vi "Input File Mode State Machine.vi"(0 "Mixed Mode Widget Requests":T9, 1 "MM In":refnum<queue>, 2 "Mixed Mode Command In":T2, 5 "Mixed Mode Widget Actions In":T8, 7 "Mixed Mode Blinkies In":T7, 13 "MixedModeStates In":T1=enum."Idle") -> (4 "Mixed Mode Widget Approval":T9, 6 "Mixed Mode Widget Actions Out":T8, 8 "Mixed Mode Blinkies Out":T7, 12 "MM Out":refnum<queue>)   [LabVIEW 2009]
uses:
  Mixed Mode Widget Requests.ctl
  Accepted or Declined.ctl
  Mixed Mode Widget State.ctl
  Messages/Mixed Mode Command.ctl
  Mixed Mode Command Action.ctl
  Ramp Time Tuple.ctl
  Target Data.ctl
  Data Access Objects/Metadata/LBCB Space.ctl
  Mixed Mode Blinkies.ctl
  Mixed Mode States.ctl
  Target Pattern.ctl
  Step DAO Actions.ctl
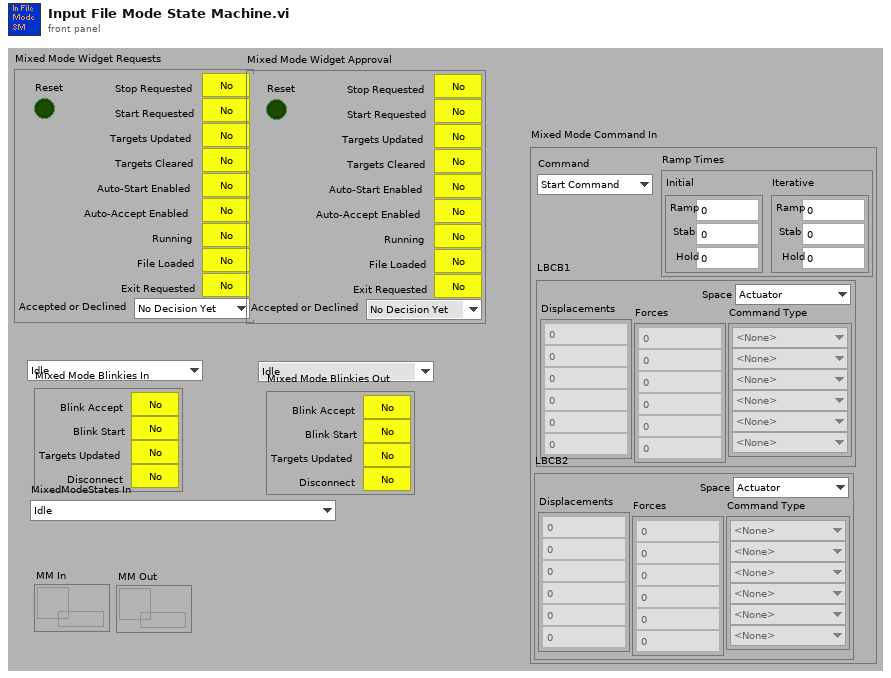
[diagram p1: front panel]
types:
  T1 = typedef "Mixed Mode States.ctl" = enum16{"Init", "Wait For DAQ", "Idle", "Start Initial Position", "Initial Position", "Start Initial Ramp", "Run Initial Ramp", "Start Iterative Stage", "Convergence Check", "Update Stiffness Jacobian", "Update Command", "Start Iterative Ramp", "Run Iterative Ramp", "Start Iterative Stabilize", "Iterative Stabilize", "Start Iterative Holding", "Iterative Holding", "Start Stabilize", "Stabilize", "Start Hold", "Holding", "Done", "Aborting", "Exit", "Nop"}
  T2 = typedef "Mixed Mode Command.ctl" = cluster{"Command":T3, "Ramp Times":cluster{"Initial":T4, "Iterative":T4}, "LBCB1":T5, "LBCB2":T5}
  T3 = typedef "Mixed Mode Command Action.ctl" = enum16{"Start Command", "Stop", "Exit", "No Op", "Start Acquisition", "Measure Initial Position"}
  T4 = typedef "Ramp Time Tuple.ctl" = cluster{"Ramp":dbl, "Stab":dbl, "Hold":dbl}
  T5 = typedef "Target Data.ctl" = cluster{"Displacements":dbl[], "Command Type":enum16{"<None>", "Displacement", "Force"}[], "Forces":dbl[], "Space":T6}
  T6 = typedef "LBCB Space.ctl" = enum16{"Actuator", "Cartesian"}
  T7 = typedef "Mixed Mode Blinkies.ctl" = cluster{"Blink Accept":bool, "Blink Start":bool, "Targets Updated":bool, "Disconnect":bool}
  T8 = typedef "Mixed Mode Widget State.ctl" = enum16{"Idle", "Auto Start", "Wait for Start", "Start", "Wait for Hold", "Waiting for Done", "Step Completed", "Limit Fault", "Stop", "Abort", "Clear Targets", "Reset", "Steps Loaded", "Paused", "Steps Available", "Load Step", "Connected", "Disconnecting", "Wait for Proposal", "Auto Accept", "Wait for Accept", "Accept", "Decline", "Wait for Execute", "Unknown", "Exit"}
  T9 = typedef "Mixed Mode Widget Requests.ctl" = cluster{"Start Requested":bool, "Targets Updated":bool, "Targets Cleared":bool, "Stop Requested":bool, "Auto-Start Enabled":bool, "Auto-Accept Enabled":bool, "Accepted or Declined":T10, "Running":bool, "File Loaded":bool, "Reset":bool, "Exit Requested":bool}
  T10 = typedef "Accepted or Declined.ctl" = enum16{"No Decision Yet", "Accepted", "Declined"}
  T11 = typedef "Target Pattern.ctl" = enum16{"Clear Targets", "Reset Targets to Zero", "Displacements Only", "Rotations Only", "Displacements & Rotations", "Forces Only", "Moments Only", "Forces & Moments"}
  T12 = typedef "Step DAO Actions.ctl" = enum16{"Init", "Set", "Get", "Reset Count"}
  T13 = typedef "Target.ctl" = cluster{"LBCB Number":T14, "DOF Vectors":enum16{" ", "Dx", "Dy", "Dz", "Rx", "Ry", "Rz", "Fx", "Fy", "Fz", "Mx", "My", "Mz"}, "Amount":dbl}
  T14 = typedef "LBCB Number.ctl" = enum16{"LBCB1", "LBCB2"}
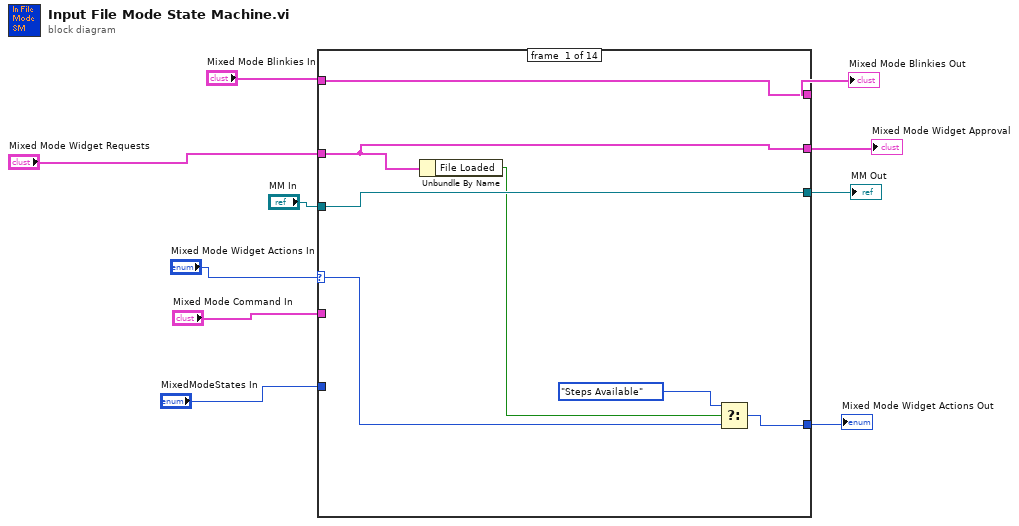
[diagram p0: block diagram]
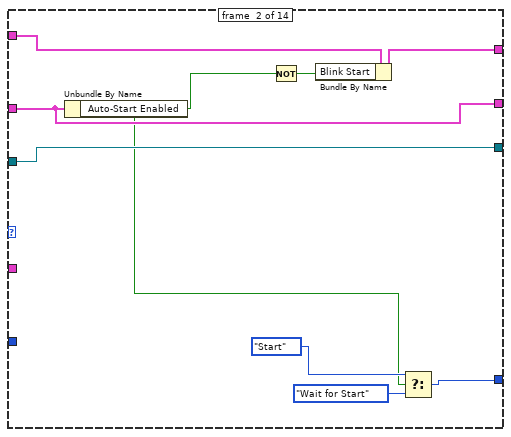
[diagram p2: hidden frame]
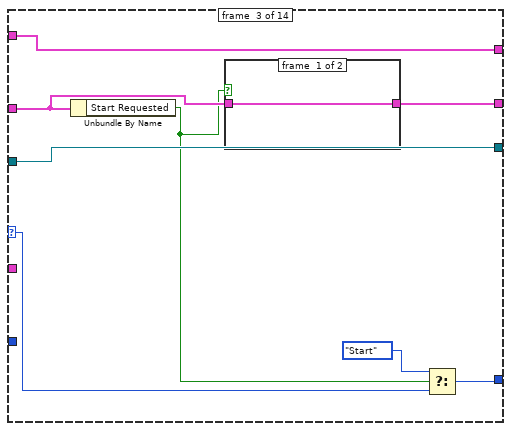
[diagram p3: hidden frame]
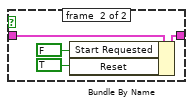
[diagram p4: hidden frame]
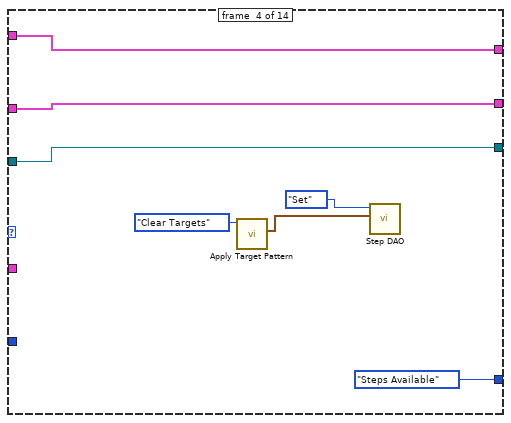
[diagram p5: hidden frame]
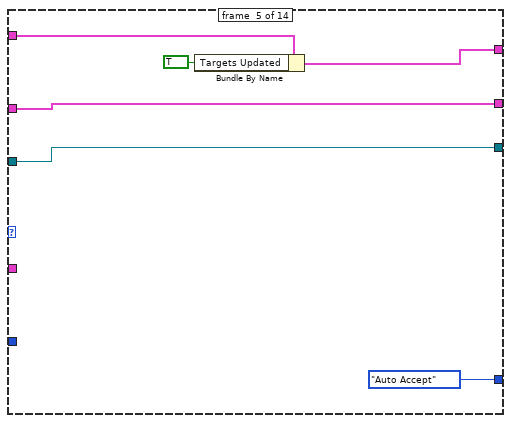
[diagram p6: hidden frame]
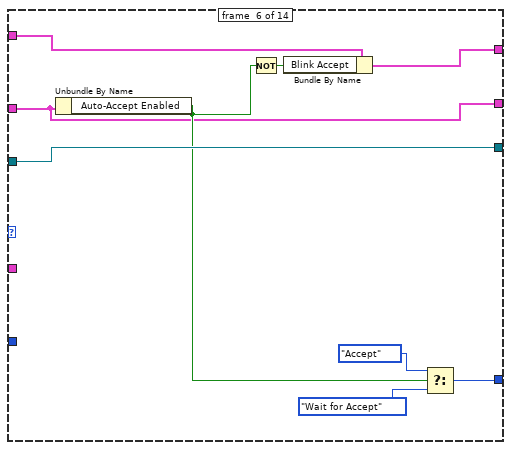
[diagram p7: hidden frame]
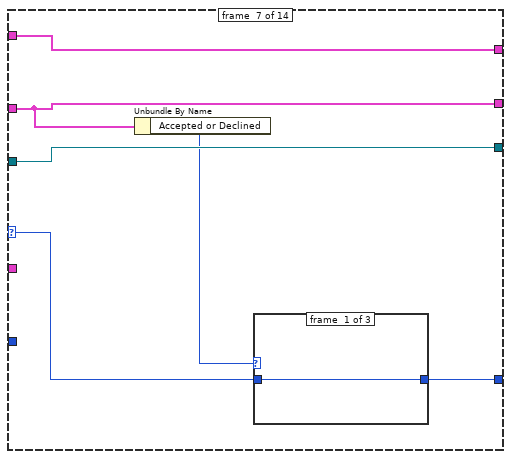
[diagram p8: hidden frame]
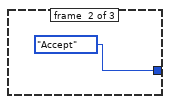
[diagram p9: hidden frame]
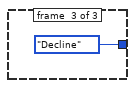
[diagram p10: hidden frame]
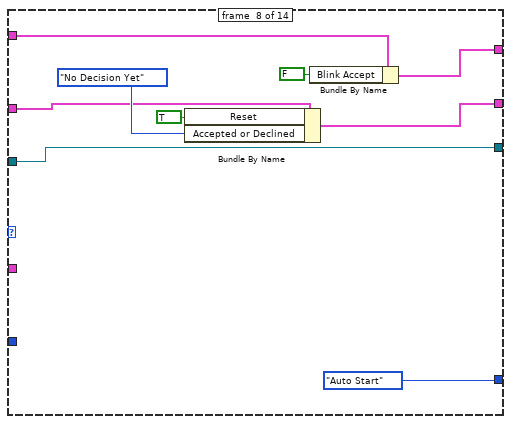
[diagram p11: hidden frame]
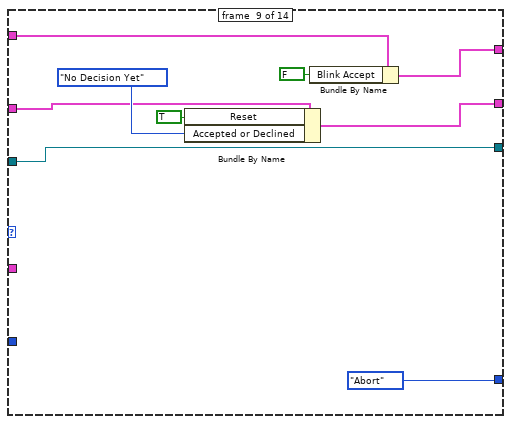
[diagram p12: hidden frame]
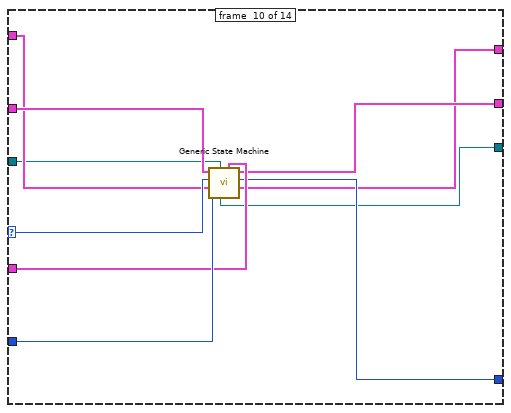
[diagram p13: hidden frame]
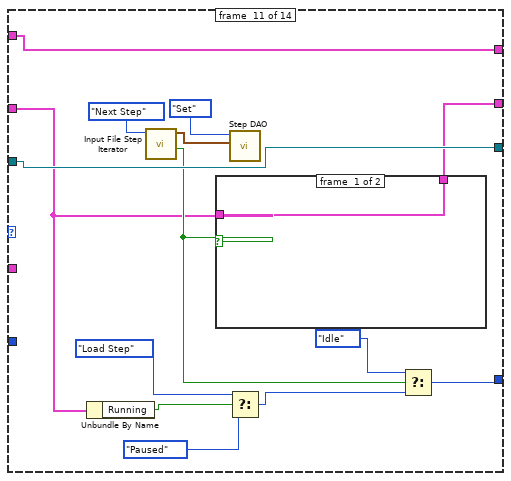
[diagram p14: hidden frame]
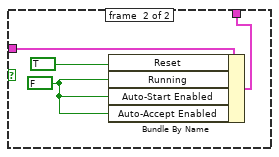
[diagram p15: hidden frame]
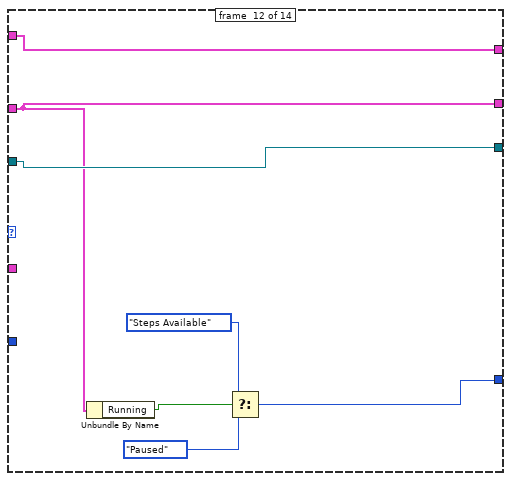
[diagram p16: hidden frame]
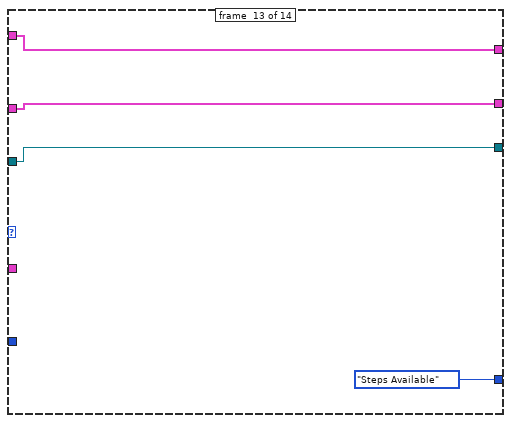
[diagram p17: hidden frame]
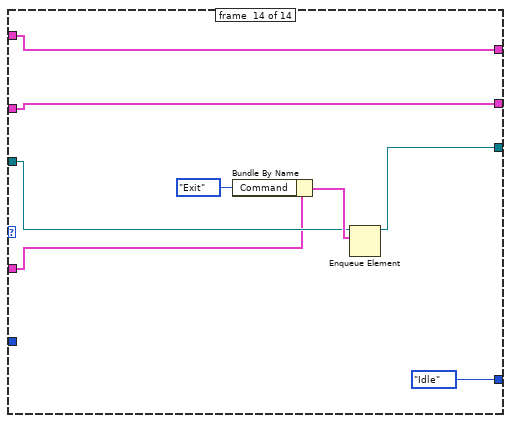
[diagram p18: hidden frame]
diagram:
  n1 = case shown="\"Steps Available\"" "Mixed Mode Widget Actions In" {
    selector: "Mixed Mode Widget Actions In" -> [w14 _ w27 _ _ _ w63 _ _ w97 _ _ _ _]
    tunnel: "Mixed Mode Widget Requests" -> [w12 w23 w30 w42 w52 w53 w62 w75 w84 w98 w100 w122 w127 w133]
    tunnel: "Mixed Mode Blinkies In" -> [w17 w26 w31 w43 w50 w61 w67 w79 w88 w96 w108 w124 w128 w134]
    tunnel: [w17 w25 w31 w43 w49 w56 w67 w78 w87 w90 w108 w124 w128 w134] -> w8
    tunnel: [w16 w20 w34 Mixed_Mode_Widget_State."Steps Available" ("Mixed Mode Widget Actions In") Mixed_Mode_Widget_State."Auto Accept" ("Mixed Mode Widget Actions In") w59 w64 Mixed_Mode_Widget_State."Auto Start" ("f") Mixed_Mode_Widget_State."Abort" ("f") w91 w109 w118 Mixed_Mode_Widget_State."Steps Available" ("f") Mixed_Mode_Widget_State."Idle" ("f")] -> w1
    tunnel: [w12 w23 w29 w42 w52 w53 w62 w74 w83 w92 w99 w122 w127 w133] -> w7
    tunnel: "Mixed Mode Command In" -> [_ _ _ _ _ _ _ _ _ w93 _ _ _ w130]
    tunnel: "MM In" -> [w13 w22 w32 w41 w51 w60 w66 w73 w82 w94 w107 w123 w126 w132]
    tunnel: [w13 w22 w32 w41 w51 w60 w66 w73 w82 w89 w107 w123 w126 w131] -> w4
    tunnel: "MixedModeStates In" -> [_ _ _ _ _ _ _ _ _ w95 _ _ _ _]
    frame #0 {
      n2 = Unbundle By Name(w12) -> ("File Loaded"=w11:bool)
      n3 = Select(t=Mixed_Mode_Widget_State."Steps Available" ("Mixed Mode Widget Actions In"), s=w11, f=w14) -> (s? t:f=w16:T8)
    }
    frame #1 {
      n4 = Unbundle By Name(w23) -> ("Auto-Start Enabled"=w19:bool)
      n5 = Not(x=w19) -> (.not. x?=w24:bool)
      n6 = Bundle By Name(cluster=w26, "Blink Start"=w24) -> (w25:T7)
      n7 = Select(t=Mixed_Mode_Widget_State."Start" ("Mixed Mode Widget Actions In"), s=w19, f=Mixed_Mode_Widget_State."Wait for Start") -> (s? t:f=w20:T8)
    }
    frame #2 {
      n8 = Unbundle By Name(w30) -> ("Start Requested"=w28:bool)
      n9 = case shown="False" w28 {
        tunnel: w30 -> [w35 w39]
        tunnel: [w35 w38] -> w29
        frame #0 {
        }
        frame #1 {
          n10 = Bundle By Name(cluster=w39, "Start Requested"=FALSE, "Reset"=TRUE) -> (w38:T9)
        }
      }
      n11 = Select(t=Mixed_Mode_Widget_State."Start", s=w28, f=w27) -> (s? t:f=w34:T8)
    }
    frame #3 {
      n12 = call "Apply Target Pattern.vi"("Target Pattern"=Target_Pattern."Clear Targets") -> ("Targets"=w45:T13[])  [unwired: 1 in, 9 out]
      n13 = call "Step DAO.vi"("Step In"=w45, "Step DAO Actions"=Step_DAO_Actions."Set") -> ()  [unwired: 2 in, 8 out]
    }
    frame #4 {
      n14 = Bundle By Name(cluster=w50, "Targets Updated"=TRUE) -> (w49:T7)
    }
    frame #5 {
      n15 = Unbundle By Name(w53) -> ("Auto-Accept Enabled"=w54:bool)
      n16 = Not(x=w54) -> (.not. x?=w55:bool)
      n17 = Bundle By Name(cluster=w61, "Blink Accept"=w55) -> (w56:T7)
      n18 = Select(t=Mixed_Mode_Widget_State."Accept" ("Mixed Mode Widget Actions In"), s=w54, f=Mixed_Mode_Widget_State."Wait for Accept") -> (s? t:f=w59:T8)
    }
    frame #6 {
      n19 = Unbundle By Name(w62) -> ("Accepted or Declined"=w65:T10)
      n20 = case shown="\"No Decision Yet\"" w65 {
        tunnel: [w68 Mixed_Mode_Widget_State."Accept" ("f") Mixed_Mode_Widget_State."Decline" ("f")] -> w64
        tunnel: w63 -> [w68 _ _]
        frame #0 {
        }
        frame #1 {
        }
        frame #2 {
        }
      }
    }
    frame #7 {
      n21 = Bundle By Name(cluster=w75, "Reset"=TRUE, "Accepted or Declined"=Accepted_or_Declined."No Decision Yet") -> (w74:T9)
      n22 = Bundle By Name(cluster=w79, "Blink Accept"=FALSE) -> (w78:T7)
    }
    frame #8 {
      n23 = Bundle By Name(cluster=w84, "Reset"=TRUE, "Accepted or Declined"=Accepted_or_Declined."No Decision Yet") -> (w83:T9)
      n24 = Bundle By Name(cluster=w88, "Blink Accept"=FALSE) -> (w87:T7)
    }
    frame #9 {
      n25 = call "Generic State Machine.vi"("Mixed Mode Command In"=w93, "MM In"=w94, "MixedModeStates In"=w95, "Mixed Mode Blinkies In"=w96, "Mixed Mode Widget Actions In"=w97, "Mixed Mode Widget Requests"=w98) -> ("Mixed Mode Blinkies Out"=w90:T7, "Mixed Mode Widget Actions Out"=w91:T8, "Mixed Mode Widget Approval"=w92:T9, "MM Out"=w89:refnum<queue>)  [unwired: 2 out]
    }
    frame #10 {
      n26 = Unbundle By Name(w100) -> ("Running"=w105:bool)
      n27 = call "Input File Step Iterator.vi"("Input File Step Actions"=enum16{"Load", "Next Step", "Reset"}."Next Step") -> ("End of Input File"=w101:bool, "Next Step"=w111:T13[])  [unwired: 3 in, 6 out]
      n28 = case shown="True" w101 {
        tunnel: w100 -> [w113 w117]
        tunnel: [w113 w116] -> w99
        frame #0 {
        }
        frame #1 {
          w114 = FALSE ("File Loaded")
          n29 = Bundle By Name(cluster=w117, "Reset"=TRUE, "Running"=w114, "Auto-Start Enabled"=w114, "Auto-Accept Enabled"=w114) -> (w116:T9)
        }
      }
      n30 = call "Step DAO.vi"("Step In"=w111, "Step DAO Actions"=Step_DAO_Actions."Set") -> ()  [unwired: 2 in, 8 out]
      n31 = Select(t=Mixed_Mode_Widget_State."Load Step" ("Mixed Mode Widget Actions In"), s=w105, f=Mixed_Mode_Widget_State."Paused") -> (s? t:f=w104:T8)
      n32 = Select(t=Mixed_Mode_Widget_State."Idle" ("f"), s=w101, f=w104) -> (s? t:f=w109:T8)
    }
    frame #11 {
      n33 = Unbundle By Name(w122) -> ("Running"=w120:bool)
      n34 = Select(t=Mixed_Mode_Widget_State."Steps Available" ("Mixed Mode Widget Actions In"), s=w120, f=Mixed_Mode_Widget_State."Paused") -> (s? t:f=w118:T8)
    }
    frame #12 {
    }
    frame #13 {
      n35 = Bundle By Name(cluster=w130, "Command"=Mixed_Mode_Command_Action."Exit") -> (w136:T2)
      n36 = Enqueue Element(queue=w132, element=w136) -> (queue out=w131:refnum<queue>)  [unwired: 1 in, 3 out]
    }
  }
  "Mixed Mode Widget Approval" <- w7
  "Mixed Mode Widget Actions Out" <- w1
  "MM Out" <- w4
  "Mixed Mode Blinkies Out" <- w8
